vi "Hot_Wire_Setup.vi"(1 "XW?":bool, 2 "Setup String":string) -> (0 "Output string":string="\rBridge 1\tNewcastle Bridge\rProbe type\t\rWire ID\t\rOverheat ratio 1\t0.500000\rGain 1\t0.000000\rLP Filter Hz 1\t0.000000\r")   [LabVIEW 2022 SP3]
uses:
  Controls/Metal_Type.ctl
  Controls/ok_button.ctl
  File/Setup_Filetype.ctl
panel:
  in  "Wire ID number":string
  in  "Probe type":u16(ring) items=["P01 (Straight, plated)", "P05 (Boundary, plated)", "P11 (Straight, miniature)", "P12 (Slant, miniature)", "P14 (Bent, miniature)", "P31 (Thermo)", "P51(Dual slant, plated)", "P51/120 (Dual slant, plated)", "P53(BL Dual slant, plated)", "P61 (Dual slant, min)", "P62 (Dual Cross, Min)", "P64 (Cross bent Min)", "P76 (Straight, temp. comp.)", "R61 (Dual Parallel, film)"]
  in  "Edit Probe Types":bool
  in  "Edit Bridge Types":bool
  in  "Ok":T1
  in  "Instrument setup":T3(array[cluster])=[{"Gain"=0.0, "LP Filter Hz"=0, "Bridge"=4, "Overheat ratio"=0.5, "Wire"="", "Offset Voltage"=0.0, "Metal Type"=enum."Tungsten"}] {"Offset Voltage" min=0.0 max=10.0 format="%#.3f"; "Overheat ratio" min=0.5 max=0.99 format="%.2f"; "Bridge" items=["DISA 56 C14", "DISA 56 C16", "DISA 56 C17", "Newcastle Bridge", "PSI 6110", "Mini CTA"]; "Gain" min=1.0 max=100.0 format="%.2f"}
  # "Rhot-Rcold\n   Rcold"
  # "V=Gain(E-Offset)"
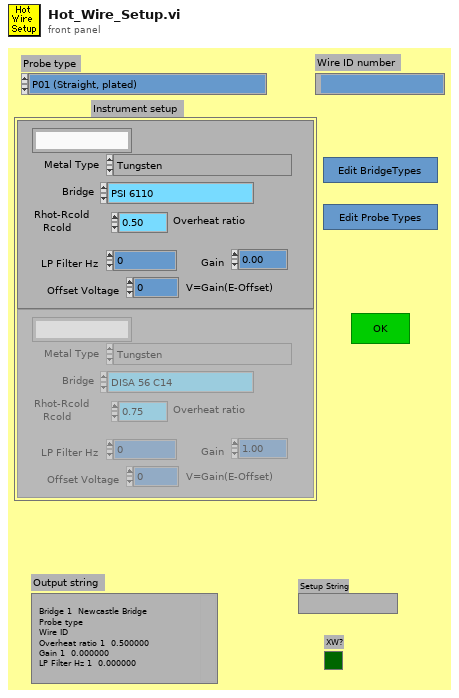
[diagram p1: front panel]
types:
  T1 = typedef "ok_button.ctl" = bool
  T2 = typedef "Metal_Type.ctl" = enum16{"Tungsten", "Platinum", "Platinum-plated Tungsten"}
  T3 = cluster{"Gain":dbl, "LP Filter Hz":i32, "Bridge":u16, "Overheat ratio":dbl, "Wire":string, "Offset Voltage":dbl, "Metal Type":T2}[]
  T4 = typedef "Setup_Filetype.ctl" = enum16{"Measurement Setups", "Calibration Setups", "General", "Results File Plotter Setups", "Speed Calib Tweaks"}
  T5 = cluster{"Gain":dbl, "LP Filter Hz":i32, "Bridge":u16, "Overheat ratio":dbl, "Wire":string, "Offset Voltage":dbl, "Metal Type":T2}
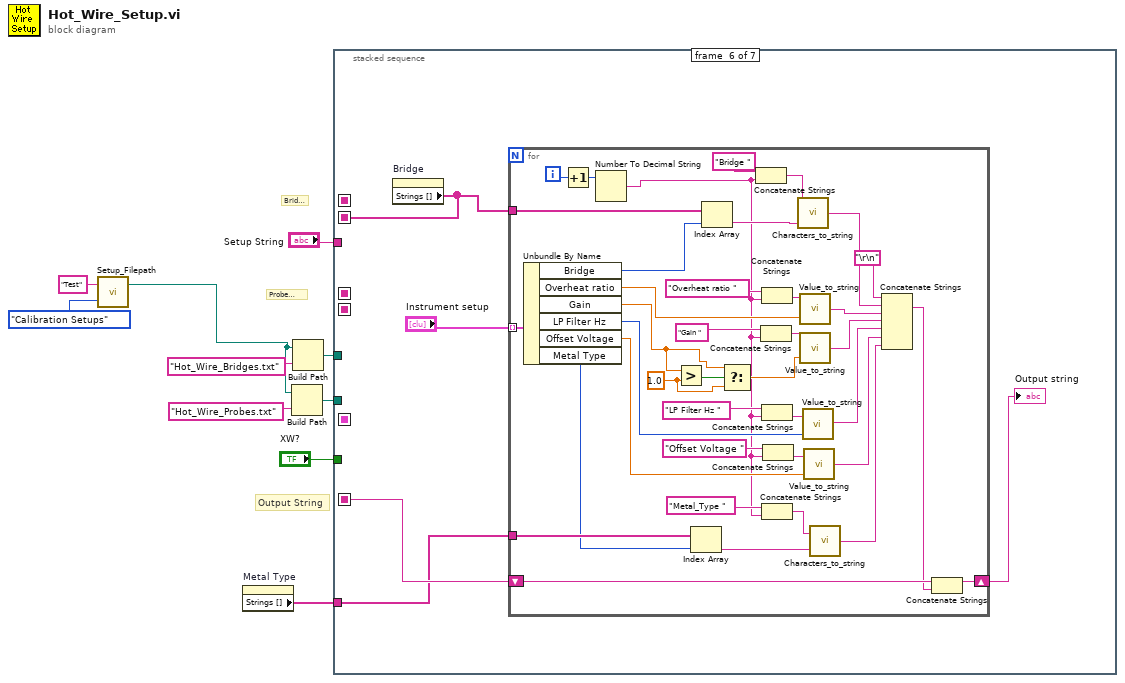
[diagram p0: block diagram]
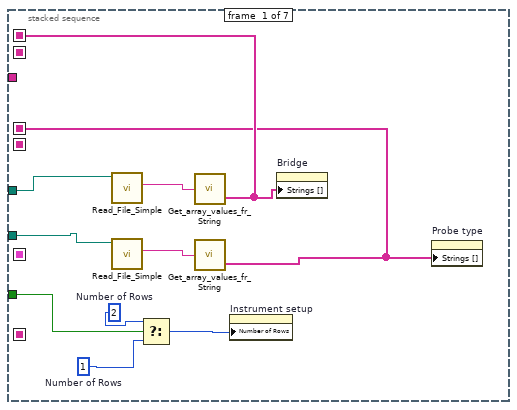
[diagram p2: hidden frame]
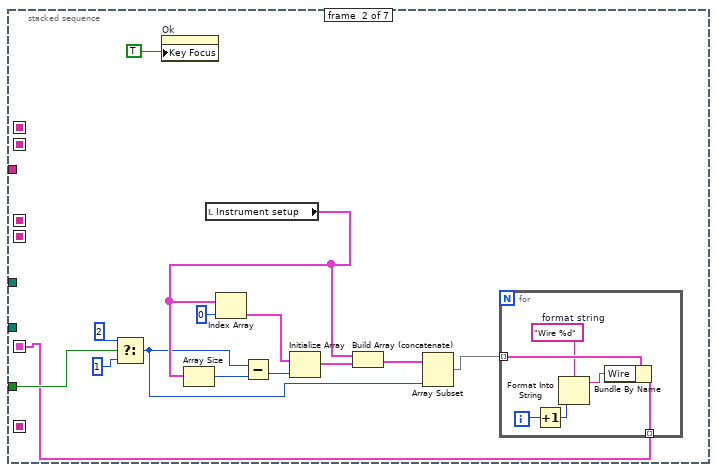
[diagram p3: hidden frame]
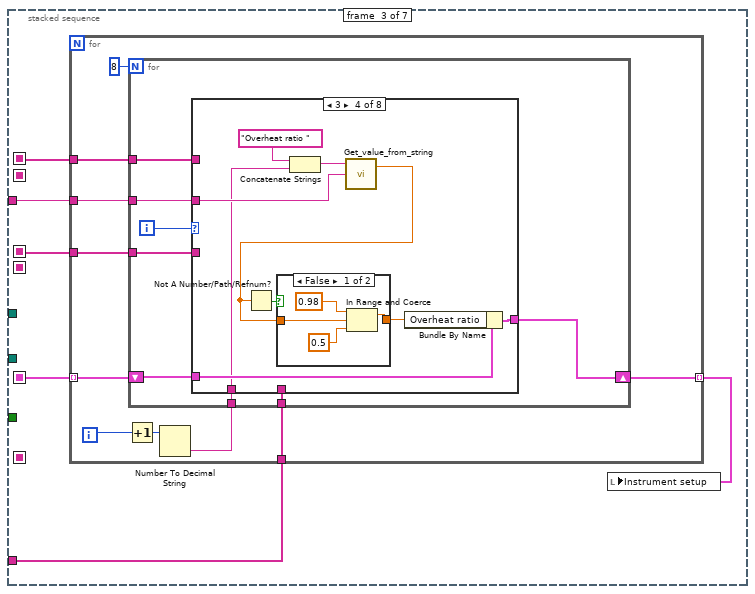
[diagram p4: hidden frame]
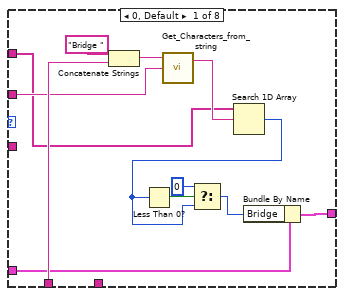
[diagram p5: hidden frame]
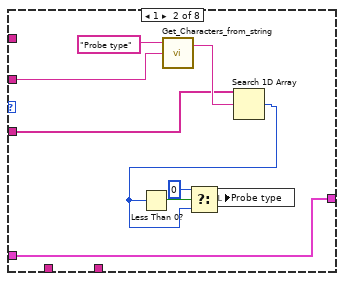
[diagram p6: hidden frame]
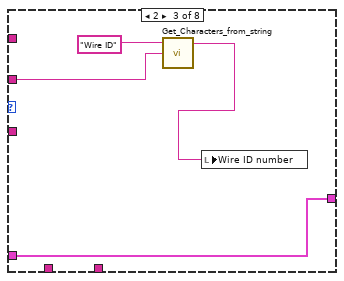
[diagram p7: hidden frame]
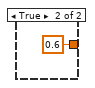
[diagram p8: hidden frame]
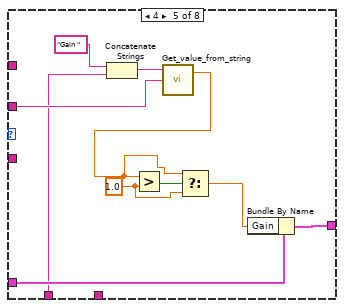
[diagram p9: hidden frame]
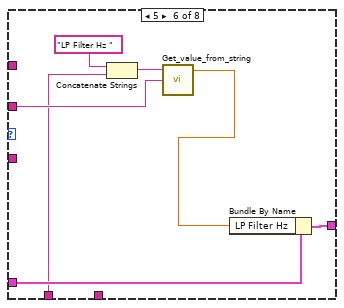
[diagram p10: hidden frame]
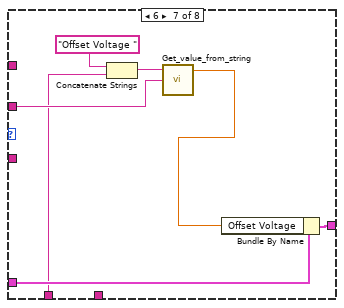
[diagram p11: hidden frame]
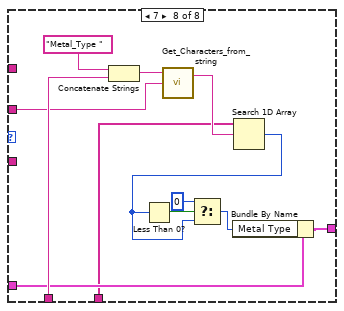
[diagram p12: hidden frame]
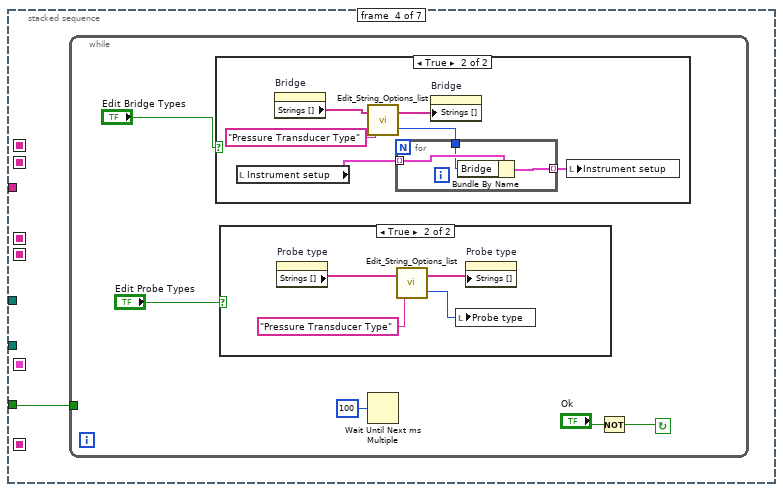
[diagram p13: hidden frame]
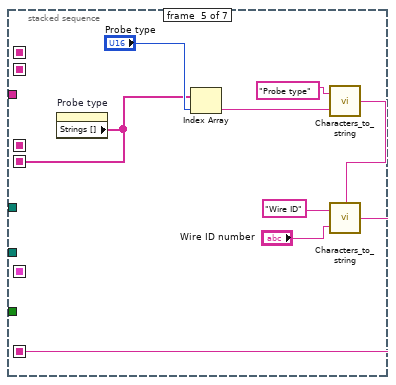
[diagram p16: hidden frame]
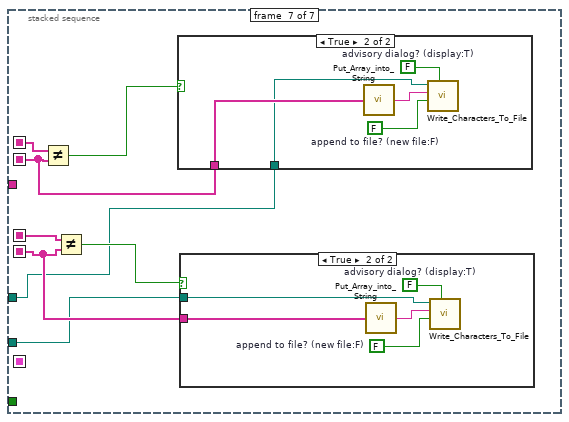
[diagram p17: hidden frame]
diagram:
  # "Probe types"
  # "Bridges"
  # "Output String"
  n1 = call "Setup_Filepath.vi"("Setup File Type"=Setup_Filetype."Calibration Setups", "Filename in"="Test") -> ("Directory"=w1:path)  [unwired: 1 out]
  n2 = property on="Metal Type" class="Enum (strict)"() -> ("Strings []"=w4:string[])  [unwired: 2 in, 2 out]
  n3 = Build Path(base path=w1, name or relative path="Hot_Wire_Probes.txt") -> (appended path=w5:path)
  n4 = Build Path(base path=w1, name or relative path="Hot_Wire_Bridges.txt") -> (appended path=w7:path)
  n5 = stacked-sequence {
    seq-local: [_ w22 _ _ _ _ _] -> [_ _ w46 _ _ _ _]
    seq-local: [_ _ _ _ w159 _ _] -> [_ _ _ _ _ w170 _]
    seq-local: [w18 _ _ _ _ _ _] -> [_ _ w42 _ _ _ w218]
    seq-local: [w15 _ _ _ _ _ _] -> [_ _ w43 _ _ _ w215]
    seq-local: [_ _ _ _ _ w171 _] -> [_ _ _ _ _ _ w216]
    seq-local: [_ _ _ _ w163 _ _] -> [_ _ _ _ _ _ w214]
    tunnel: "XW?" -> [w14 w28 _ w140 _ _ _]
    tunnel: "Setup String" -> [_ _ w44 _ _ _ _]
    tunnel: w7 -> [w19 _ _ _ _ _ w211]
    tunnel: w5 -> [w16 _ _ _ _ _ w212]
    tunnel: w4 -> [_ _ w41 _ _ w167 _]
    frame #0 {
      w11 = u32 1  # Number of Rows
      w12 = u32 2  # Number of Rows
      n6 = call "Read_File_Simple.vi"("Filename"=w19) -> ("string"=w20:string)  [unwired: 2 in, 7 out]
      n7 = call "Read_File_Simple.vi"("Filename"=w16) -> ("string"=w17:string)  [unwired: 2 in, 7 out]
      n8 = Select(t=w12, s=w14, f=w11) -> (s? t:f=w13:u32)
      n9 = call "Get_array_values_fr_String.vi"("String Value"=w20) -> ("String array"=w18:string[])  [unwired: 1 out]
      n10 = call "Get_array_values_fr_String.vi"("String Value"=w17) -> ("String array"=w15:string[])  [unwired: 1 out]
      n11 = property on="Instrument setup" class="Arr (strict)"("Number of Rows"=w13) -> ()  [unwired: 2 in, 2 out]
      n12 = property on="Bridge" class="Ring (strict)"("Strings []"=w18) -> ()  [unwired: 2 in, 2 out]
      n13 = property on="Probe type" class="Ring (strict)"("Strings []"=w15) -> ()  [unwired: 2 in, 2 out]
    }
    frame #1 {
      n14 = Select(t=2, s=w28, f=1) -> (s? t:f=w24:i32)
      n15 = property on="Ok" class="Bool"("Key Focus"=TRUE) -> ()  [unwired: 2 in, 2 out]
      n16 = local read "Instrument setup"() -> (w29:T3)
      n17 = Array Size(array=w29) -> (size(s)=w34:i32)
      n18 = Index Array(array=w29, index=0 ("Index")) -> (element=w31:T5)
      n19 = Subtract(x=w24, y=w34) -> (x-y=w33:i32)
      n20 = Initialize Array(w31, w33) -> (w30:T3)
      n21 = Build Array (concatenate)(w29, w30) -> (w25:T3)
      n22 = Array Subset(array=w25, length=w24) -> (w21:T3)  [unwired: 1 in]
      n23 = for {
        tunnel: [w40] -> w22 mode=indexing
        tunnel: w21 -> [w39] mode=indexing
        i -> [w38]
        w36 = "Wire %d"  # format string
        n24 = Increment(x=w38) -> (x+1=w37:i32)
        n25 = Format Into String(format string=w36, w37) -> (resulting string=w35:string)  [unwired: 2 in, 1 out]
        n26 = Bundle By Name(cluster=w39, "Wire"=w35) -> (w40:T5)
      }
    }
    frame #2 {
      n27 = for {
        tunnel: w46 -> [w55] mode=indexing
        tunnel: [w54] -> w45 mode=indexing
        tunnel: w44 -> [w50]
        tunnel: w42 -> [w49]
        tunnel: w43 -> [w48]
        tunnel: w41 -> [w47]
        i -> [w52]
        n28 = Increment(x=w52) -> (x+1=w53:i32)
        n29 = Number To Decimal String(number=w53) -> (decimal integer string=w51:string)  [unwired: 1 out]
        n30 = for {
          N: 8 -> [_]
          shift-right: [w60] -> w54
          shift-left: w55 -> [w63]
          tunnel: w51 -> [w62]
          tunnel: w50 -> [w61]
          tunnel: w49 -> [w59]
          tunnel: w48 -> [w58]
          tunnel: w47 -> [w57]
          i -> [w64]
          n31 = case shown="3" w64 {
            tunnel: w63 -> [w72 w78 w87 w97 w112 w119 w126 w135]
            tunnel: w62 -> [w75 _ _ w94 w109 w115 w122 w138]
            tunnel: w61 -> [w73 w85 w89 w98 w113 w120 w127 w136]
            tunnel: [w70 w78 w87 w96 w111 w118 w125 w133] -> w60
            tunnel: w59 -> [w69 _ _ _ _ _ _ _]
            tunnel: w58 -> [_ w82 _ _ _ _ _ _]
            tunnel: w57 -> [_ _ _ _ _ _ _ w128]
            frame 0, Default {
              n32 = Concatenate Strings("Bridge ", w75) -> (w74:string)
              n33 = call "Get_Characters_from_string.vi"("Input string"=w73, "Variable name"=w74) -> ("Value"=w71:string)  [unwired: 1 in, 1 out]
              n34 = Search 1D Array(1D array=w69, element=w71) -> (index of element=w66:i32)  [unwired: 1 out]
              n35 = Less Than 0?(x=w66) -> (x < 0?=w67:bool)
              n36 = Select(t=0, s=w67, f=w66) -> (s? t:f=w65:i32)
              n37 = Bundle By Name(cluster=w72, "Bridge"=w65) -> (w70:T5)
            }
            frame 1 {
              n38 = call "Get_Characters_from_string.vi"("Input string"=w85, "Variable name"="Probe type") -> ("Value"=w84:string)  [unwired: 1 in, 1 out]
              n39 = Search 1D Array(1D array=w82, element=w84) -> (index of element=w79:i32)  [unwired: 1 out]
              n40 = Less Than 0?(x=w79) -> (x < 0?=w80:bool)
              n41 = Select(t=0, s=w80, f=w79) -> (s? t:f=w77:i32)
              n42 = local write "Probe type"(w77) -> ()
            }
            frame 2 {
              n43 = call "Get_Characters_from_string.vi"("Input string"=w89, "Variable name"="Wire ID") -> ("Value"=w86:string)  [unwired: 1 in, 1 out]
              n44 = local write "Wire ID number"(w86) -> ()
            }
            frame 3 {
              n45 = Concatenate Strings("Overheat ratio ", w94) -> (w93:string)
              n46 = call "Get_value_from_string.vi"("Input string"=w98, "Variable name"=w93) -> ("Value"=w91:dbl)  [unwired: 1 in, 1 out]
              n47 = Not A Number/Path/Refnum?(number/path/refnum=w91) -> (NaN/Path/Refnum?=w90:bool)
              n48 = case shown="False" w90 {
                tunnel: [w100 0.6 ("upper limit")] -> w92
                tunnel: w91 -> [w99 _]
                frame False {
                  n49 = In Range and Coerce(upper limit=0.98, x=w99, lower limit=0.5) -> (coerced(x)=w100:dbl)  [unwired: 1 out]
                }
                frame True {
                }
              }
              n50 = Bundle By Name(cluster=w97, "Overheat ratio"=w92) -> (w96:T5)
            }
            frame 4 {
              w105 = 1.0 ("y")
              n51 = Concatenate Strings("Gain ", w109) -> (w108:string)
              n52 = call "Get_value_from_string.vi"("Input string"=w113, "Variable name"=w108) -> ("Value"=w106:dbl)  [unwired: 1 in, 1 out]
              n53 = Greater?(x=w106, y=w105) -> (0:w107:bool)
              n54 = Select(t=w106, s=w107, f=w105) -> (s? t:f=w104:dbl)
              n55 = Bundle By Name(cluster=w112, "Gain"=w104) -> (w111:T5)
            }
            frame 5 {
              n56 = Concatenate Strings("LP Filter Hz ", w115) -> (w114:string)
              n57 = call "Get_value_from_string.vi"("Input string"=w120, "Variable name"=w114) -> ("Value"=w117:dbl)  [unwired: 1 in, 1 out]
              n58 = Bundle By Name(cluster=w119, "LP Filter Hz"=w117) -> (w118:T5)
            }
            frame 6 {
              n59 = Concatenate Strings("Offset Voltage ", w122) -> (w121:string)
              n60 = call "Get_value_from_string.vi"("Input string"=w127, "Variable name"=w121) -> ("Value"=w124:dbl)  [unwired: 1 in, 1 out]
              n61 = Bundle By Name(cluster=w126, "Offset Voltage"=w124) -> (w125:T5)
            }
            frame 7 {
              n62 = Concatenate Strings("Metal_Type ", w138) -> (w137:string)
              n63 = call "Get_Characters_from_string.vi"("Input string"=w136, "Variable name"=w137) -> ("Value"=w134:string)  [unwired: 1 in, 1 out]
              n64 = Search 1D Array(1D array=w128, element=w134) -> (index of element=w130:i32)  [unwired: 1 out]
              n65 = Less Than 0?(x=w130) -> (x < 0?=w131:bool)
              n66 = Select(t=0, s=w131, f=w130) -> (s? t:f=w129:i32)
              n67 = Bundle By Name(cluster=w135, "Metal Type"=w129) -> (w133:T5)
            }
          }
        }
      }
      n68 = local write "Instrument setup"(w45) -> ()
    }
    frame #3 {
      n69 = while {
        tunnel: w140 -> [_]
        stop <- w145 continue-if-true
        n70 = case shown="True" "Edit Bridge Types" {
          frame False {
          }
          frame True {
            n71 = local read "Instrument setup"() -> (w152:T3)
            n72 = property on="Bridge" class="Ring (strict)"() -> ("Strings []"=w154:string[])  [unwired: 2 in, 2 out]
            n73 = call "Edit_String_Options_list.vi"("Channel Name"="Pressure Transducer Type", "String array"=w154) -> ("New Selection Index"=w150:i32, "String array Out"=w153:string[])
            n74 = for {
              tunnel: w152 -> [w158] mode=indexing
              tunnel: [w157] -> w151 mode=indexing
              tunnel: w150 -> [w156]
              n75 = Bundle By Name(cluster=w158, "Bridge"=w156) -> (w157:T5)
            }
            n76 = property on="Bridge" class="Ring (strict)"("Strings []"=w153) -> ()  [unwired: 2 in, 2 out]
            n77 = local write "Instrument setup"(w151) -> ()
          }
        }
        n78 = case shown="True" "Edit Probe Types" {
          frame False {
          }
          frame True {
            n79 = property on="Probe type" class="Ring (strict)"() -> ("Strings []"=w147:string[])  [unwired: 2 in, 2 out]
            n80 = call "Edit_String_Options_list.vi"("Channel Name"="Pressure Transducer Type", "String array"=w147) -> ("New Selection Index"=w146:i32, "String array Out"=w148:string[])
            n81 = local write "Probe type"(w146) -> ()
            n82 = property on="Probe type" class="Ring (strict)"("Strings []"=w148) -> ()  [unwired: 2 in, 2 out]
          }
        }
        n83 = Wait Until Next ms Multiple(millisecond multiple=u32 100) -> ()  [unwired: 1 out]
        n84 = Not(x="Ok") -> (.not. x?=w145:T1)
      }
    }
    frame #4 {
      n85 = property on="Probe type" class="Ring (strict)"() -> ("Strings []"=w163:string[])  [unwired: 2 in, 2 out]
      n86 = Index Array(array=w163, index="Probe type") -> (element=w162:string)
      n87 = call "Characters_to_string.vi"("Characters to write"=w162, "Label for characters"="Probe type") -> ("Output string"=w160:string)  [unwired: 1 in]
      n88 = call "Characters_to_string.vi"("stringIn"=w160, "Characters to write"="Wire ID number", "Label for characters"="Wire ID") -> ("Output string"=w159:string)
    }
    frame #5 {
      n89 = property on="Bridge" class="Ring (strict)"() -> ("Strings []"=w171:string[])  [unwired: 2 in, 2 out]
      n90 = for {
        shift-right: [w204] -> w169
        shift-left: w170 -> [w203]
        tunnel: "Instrument setup" -> [w191] mode=indexing
        tunnel: w171 -> [w190]
        tunnel: w167 -> [w176]
        i -> [w201]
        w181 = 1.0 ("y")
        n91 = Unbundle By Name(w191) -> ("Bridge"=w189:u16, "Overheat ratio"=w205:dbl, "Gain"=w180:dbl, "LP Filter Hz"=w209:i32, "Offset Voltage"=w185:dbl, "Metal Type"=w175:T2)
        n92 = Increment(x=w201) -> (x+1=w200:i32)
        n93 = Number To Decimal String(number=w200) -> (decimal integer string=w177:string)  [unwired: 1 out]
        n94 = Greater?(x=w180, y=w181) -> (0:w182:bool)
        n95 = Index Array(array=w176, index=w175) -> (element=w173:string)
        n96 = Index Array(array=w190, index=w189) -> (element=w206:string)
        n97 = Select(t=w180, s=w182, f=w181) -> (s? t:f=w179:dbl)
        n98 = Concatenate Strings("Bridge ", w177) -> (w198:string)
        n99 = Concatenate Strings("Gain ", w177) -> (w193:string)
        n100 = Concatenate Strings("Overheat ratio ", w177) -> (w196:string)
        n101 = Concatenate Strings("LP Filter Hz ", w177) -> (w192:string)
        n102 = Concatenate Strings("Metal_Type ", w177) -> (w174:string)
        n103 = Concatenate Strings("Offset Voltage ", w177) -> (w186:string)
        n104 = call "Characters_to_string.vi"("Characters to write"=w206, "Label for characters"=w198) -> ("Output string"=w188:string)  [unwired: 1 in]
        n105 = call "Value_to_string.vi"("Value"=w205, "Label for value"=w196) -> ("Output string"=w207:string)  [unwired: 1 in]
        n106 = call "Value_to_string.vi"("Value"=w179, "Label for value"=w193) -> ("Output string"=w208:string)  [unwired: 1 in]
        n107 = call "Value_to_string.vi"("Value"=w209, "Label for value"=w192) -> ("Output string"=w210:string)  [unwired: 1 in]
        n108 = call "Value_to_string.vi"("Value"=w185, "Label for value"=w186) -> ("Output string"=w183:string)  [unwired: 1 in]
        n109 = call "Characters_to_string.vi"("Characters to write"=w173, "Label for characters"=w174) -> ("Output string"=w172:string)  [unwired: 1 in]
        n110 = Concatenate Strings("\r\n", w188, w207, w208, w210, w183, w172) -> (w202:string)
        n111 = Concatenate Strings(w203, w202) -> (w204:string)
      }
      "Output string" <- w169
    }
    frame #6 {
      n112 = Not Equal?(x=w218, y=w216) -> (x != y?=w217:bool)
      n113 = Not Equal?(x=w215, y=w214) -> (x != y?=w213:bool)
      n114 = case shown="True" w217 {
        tunnel: w216 -> [_ w225]
        tunnel: w211 -> [_ w224]
        frame False {
        }
        frame True {
          w226 = FALSE  # append to file? (new file:F)
          w227 = FALSE  # advisory dialog? (display:T)
          n115 = call "Put_Array_into_String.vi"("String array"=w225) -> ("String Value"=w228:string)
          n116 = call "Write_Characters_To_File.vi"("file path (dialog if empty)"=w224, "advisory dialog? (display:T)"=w227, "character string"=w228, "append to file? (new file:F)"=w226) -> ()  [unwired: 1 in, 4 out]
        }
      }
      n117 = case shown="True" w213 {
        tunnel: w214 -> [_ w220]
        tunnel: w212 -> [_ w219]
        frame False {
        }
        frame True {
          w221 = FALSE  # append to file? (new file:F)
          w222 = FALSE  # advisory dialog? (display:T)
          n118 = call "Put_Array_into_String.vi"("String array"=w220) -> ("String Value"=w223:string)
          n119 = call "Write_Characters_To_File.vi"("file path (dialog if empty)"=w219, "advisory dialog? (display:T)"=w222, "character string"=w223, "append to file? (new file:F)"=w221) -> ()  [unwired: 1 in, 4 out]
        }
      }
    }
  }
